vi "ReadConfigErrorParams.vi"(7 "hardware":enum16{"CAMERA", "PMT"}(ring), 11 "configuration file path":path) -> (3 "err_params":T1)   [LabVIEW 2019]
uses:
  <vilib>/Utility/config.llb/Read Key (I32).vi
  <vilib>/Utility/config.llb/Read Key (String).vi
  <vilib>/Utility/config.llb/NI_LVConfig.lvlib
panel:
  out "errm1":string
  out "errm2":string
  out "t2":i32
  out "t1":i32
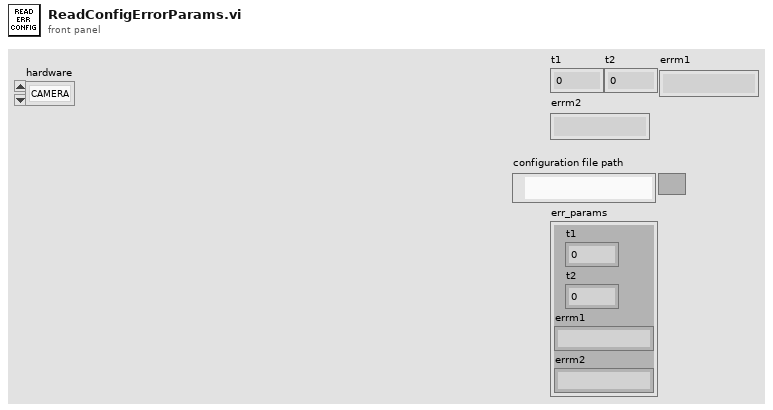
[diagram p1: front panel]
types:
  T1 = cluster{"t1":i32, "t2":i32, "errm1":string, "errm2":string}
  T2 = typedef "NI_LVConfig.lvlib/Config Data RefNum.ctl" = refnum<k1>
  T3 = cluster{"value":i32, "value":i32, "value":string, "value":string}
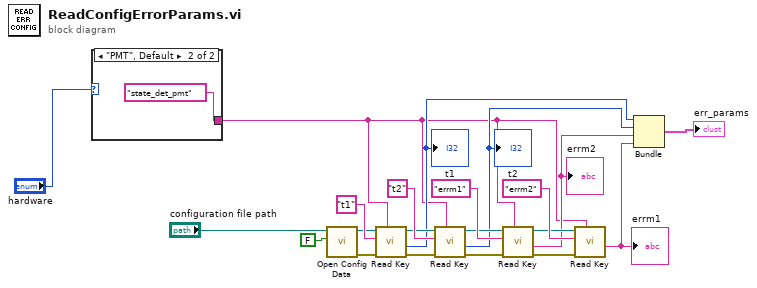
[diagram p0: block diagram]
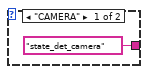
[diagram p2: hidden frame]
diagram:
  n1 = case shown="\"PMT\", Default" "hardware" {
    tunnel: ["state_det_camera" "state_det_pmt"] -> w2
    frame "CAMERA" {
    }
    frame "PMT", Default {
    }
  }
  n2 = call <vilib>:"Open Config Data.vi"("create file if necessary (T)"=FALSE, "configuration file path"="configuration file path") -> ("error out"=w17:errorcluster, "refnum"=w18:T2)  [unwired: 7 in, 1 out]
  n3 = call-poly <vilib>:"Read Key.vi"("section"=w2, "error in (no error)"=w17, "key"="t1", "refnum"=w18) -> ("error out"=w13:errorcluster, "value"=w7:i32, "refnum out"=w10:T2)  [unwired: 4 in, 1 out]
  "t1" <- w7
  n4 = call-poly <vilib>:"Read Key.vi"("section"=w2, "error in (no error)"=w13, "key"="t2", "refnum"=w10) -> ("error out"=w12:errorcluster, "value"=w6:i32, "refnum out"=w9:T2)  [unwired: 4 in, 1 out]
  "t2" <- w6
  n5 = call-poly <vilib>:"Read Key.vi"("section"=w2, "error in (no error)"=w12, "key"="errm1", "refnum"=w9) -> ("error out"=w11:errorcluster, "value"=w5:string, "refnum out"=w8:T2)  [unwired: 4 in, 1 out]
  "errm2" <- w5
  n6 = call-poly <vilib>:"Read Key.vi"("section"=w2, "error in (no error)"=w11, "key"="errm2", "refnum"=w8) -> ("value"=w4:string)  [unwired: 4 in, 3 out]
  "errm1" <- w4
  n7 = Bundle("value"=w7, "value"=w6, "value"=w5, "value"=w4) -> (→"err_params":T3)  [unwired: 1 in]
